vi "Efficiency and Load regulation UI.vi"() -> ()   [LabVIEW 2021]
panel:
  in  "MeasGraphs":T1(tab)
  out "EfficiencyGraph":T2(graph)
  out "LoadRegulationGraph(V/A)":T3(graph)
  out "LoadRegulationGraph(%)":T4(graph)
  out "Load voltage deviation":dbl[](array[numeric])
  out "Load voltages":dbl[](array[numeric])
  out "Efficiency":dbl[](array[numeric])
  out "Load currents":dbl[](array[numeric])
  in  "Source resource name":string caption="RESOURCE NAME"
  in  "Load resource name":string caption="RESOURCE NAME"
  in  "Load Current":dbl
  in  "Source Voltage":dbl
  in  "Load sense":i32(ring)=1009 caption="SENSE" items=["Local"=1008, "Remote"=1009]
  in  "Source sense":i32(ring)=1009 caption="SENSE" items=["Local"=1008, "Remote"=1009]
  out "Status":string
  in  "ELOADResourceName":refnum<k15> caption="RESOURCE NAME"
  in  "PPSResourceName":refnum<k15> caption="RESOURCE NAME"
  in  "DUT setup time":dbl=1.0 caption="DUT SETUP TIME" format="%#_6ps"
  in  "Aperture time":dbl=0.005 caption="APERTURE TIME" format="%#_6ps"
  in  "Source delay":dbl=0.005 caption="SOURCE DELAY" format="%#_6ps"
  in  "Load voltage limit range":dbl=6.0 caption="VOLTAGE LIMIT RANGE" format="%#_6pV"
  in  "Source current limit":dbl=25.0 caption="CURRENT LIMIT" format="%#_6pA"
  in  "Source maximum power":dbl=300.0 caption="MAXIMUM POWER" format="%#_6pW"
  in  "Load configuration":string="Load configuration"
  in  "Source configuration":string="Source configuration"
  in  "Measurement settings":string="Measurement settings"
  in  "Nominal output voltage":dbl=3.3 caption="NOMINAL OUTPUT VOLTAGE" format="%#_6pV"
  in  "Mode of operation":T5(ring)=enum."Perform measurement" caption="MODE OF OPERATION"
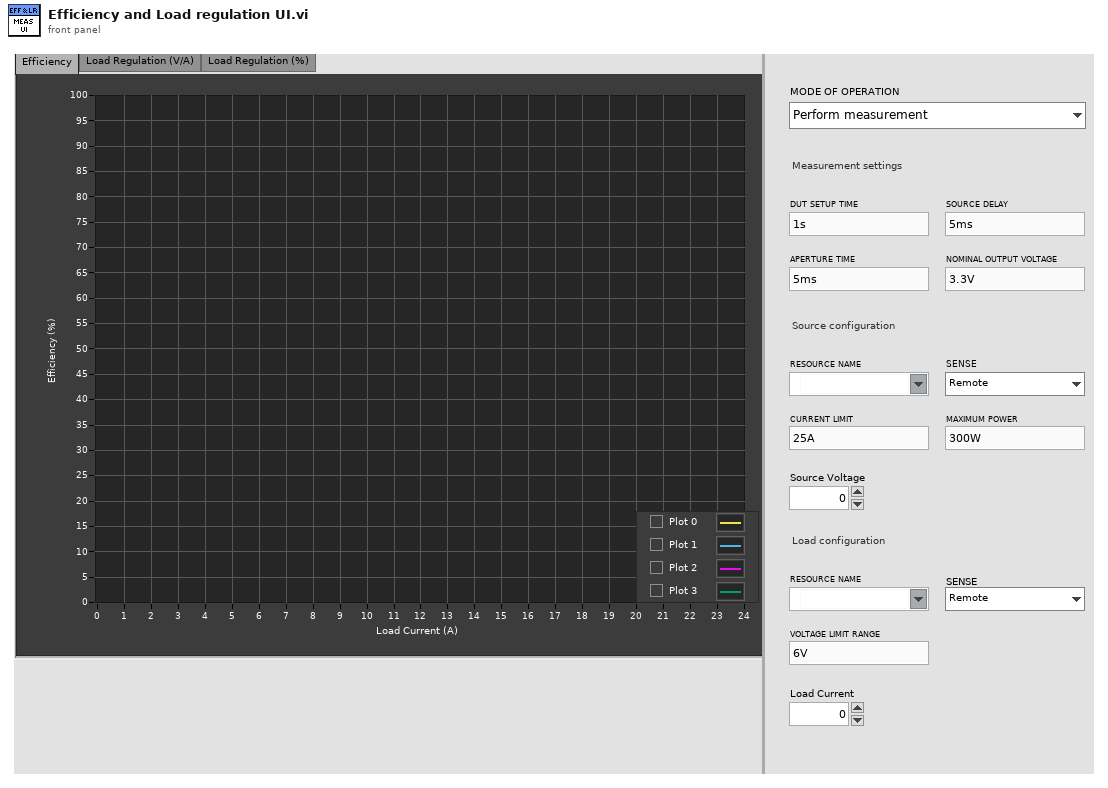
[diagram p1: front panel]
types:
  T1 = enum32{"Efficiency", "Load Regulation (V/A)", "Load Regulation (%)", "Hidden Controls"}
  T2 = cluster{"Load currents":dbl[], "Efficiency":dbl[]}
  T3 = cluster{"Load currents":dbl[], "Load voltages":dbl[]}
  T4 = cluster{"Load currents":dbl[], "Load voltage deviation":dbl[]}
  T5 = enum32{"Power on the DUT", "Perform measurement", "Power off the DUT"}
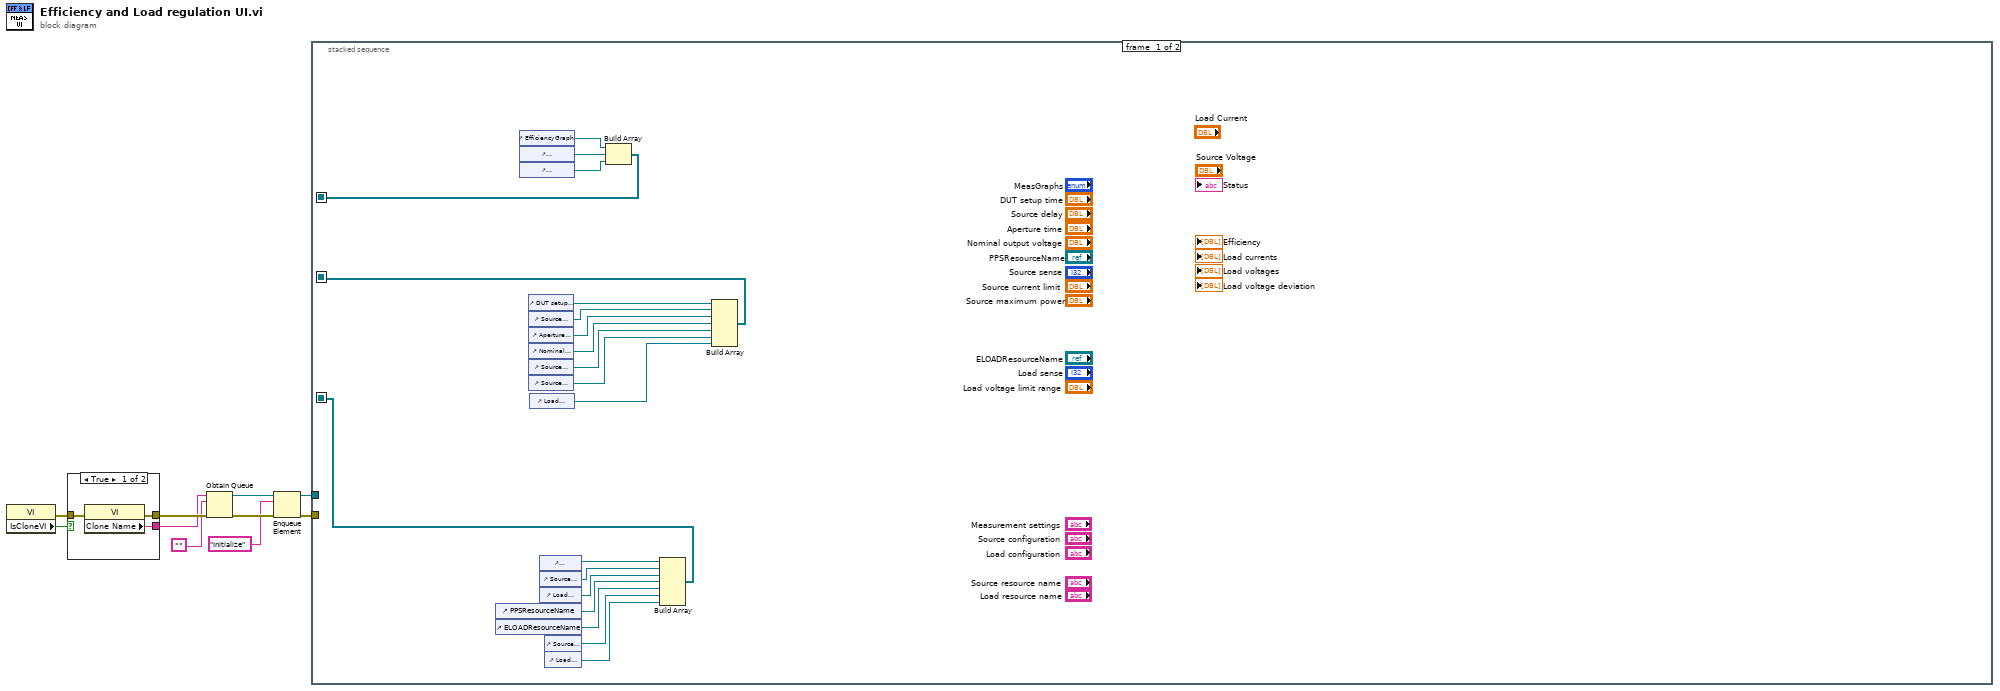
[diagram p0: block diagram]
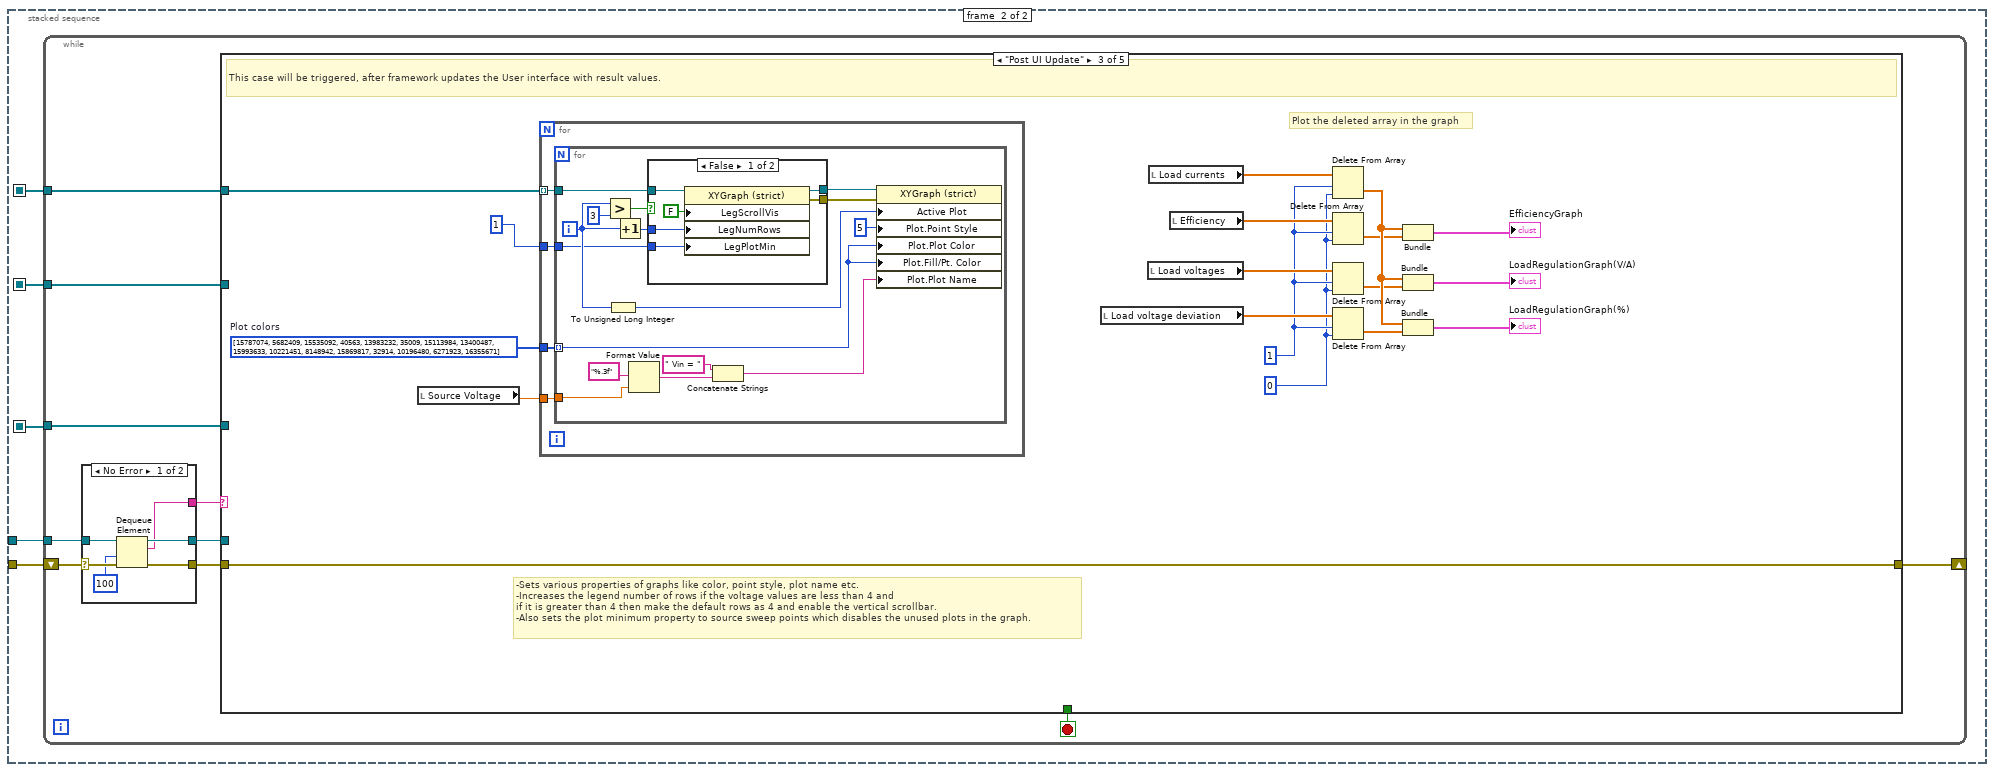
[diagram p2: hidden frame]
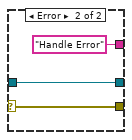
[diagram p3: hidden frame]
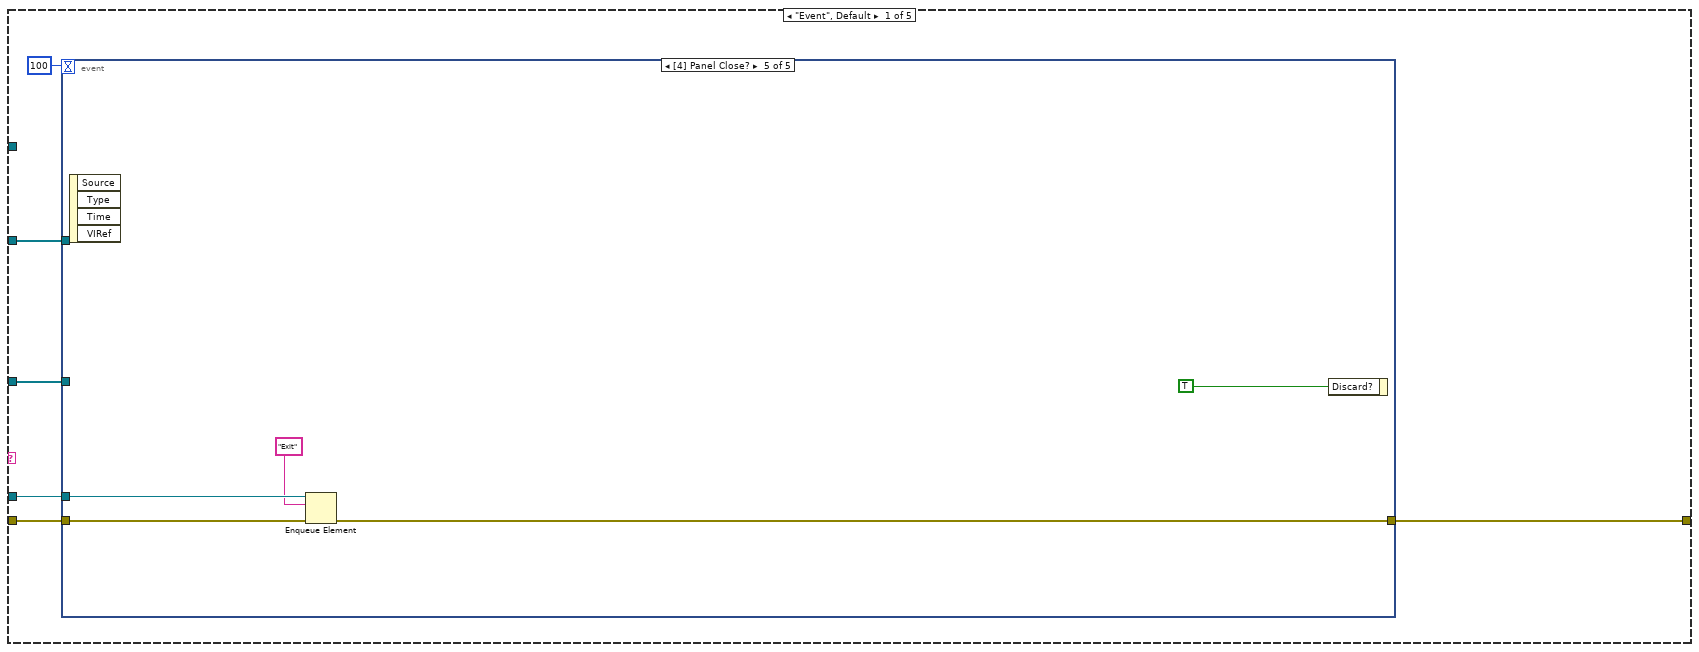
[diagram p4: hidden frame]
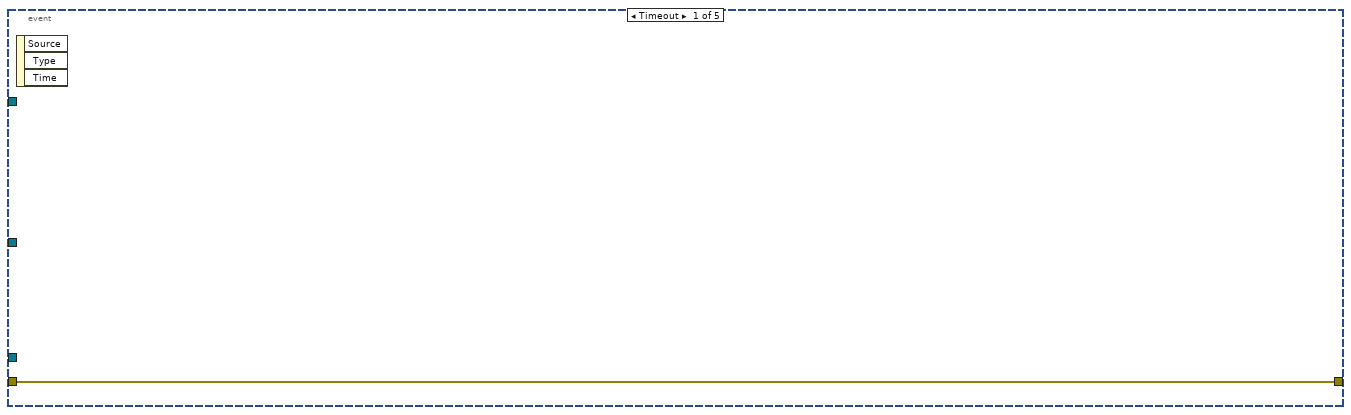
[diagram p5: hidden frame]
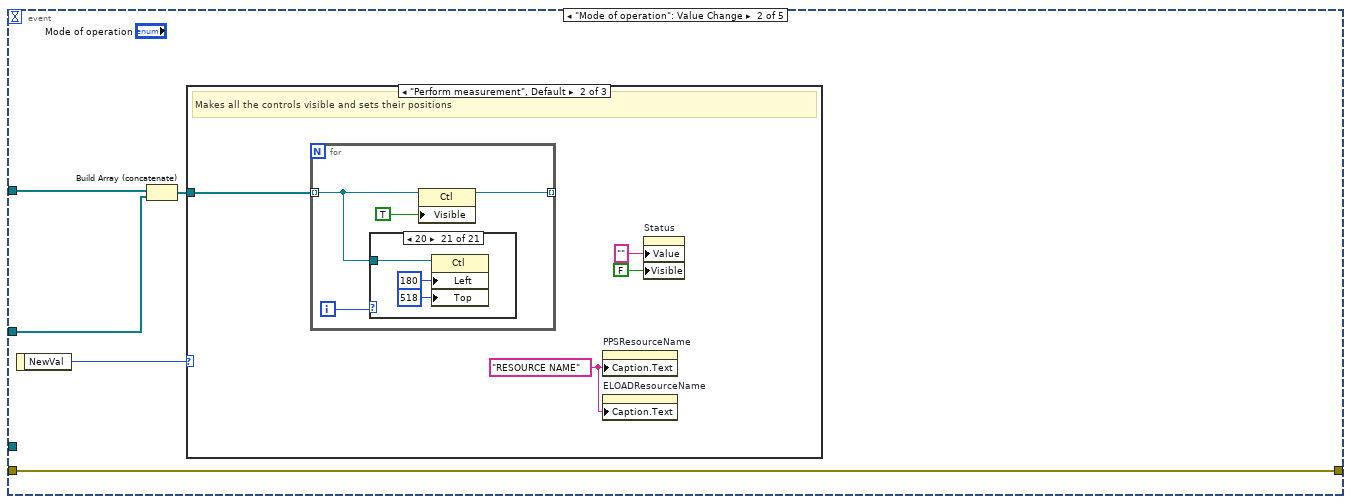
[diagram p6: hidden frame]
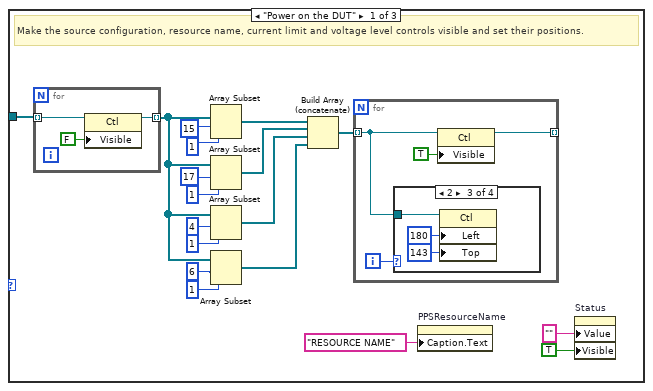
[diagram p7: hidden frame]
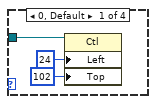
[diagram p8: hidden frame]
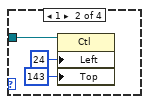
[diagram p9: hidden frame]
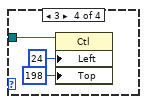
[diagram p10: hidden frame]
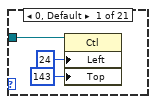
[diagram p11: hidden frame]
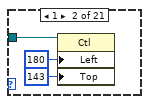
[diagram p12: hidden frame]
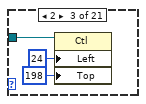
[diagram p13: hidden frame]
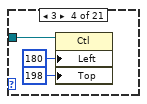
[diagram p14: hidden frame]
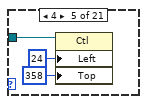
[diagram p15: hidden frame]
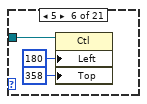
[diagram p16: hidden frame]
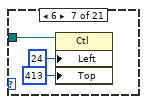
[diagram p17: hidden frame]
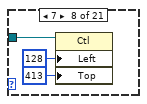
[diagram p18: hidden frame]
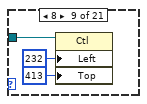
[diagram p19: hidden frame]
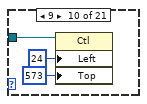
[diagram p20: hidden frame]
diagram:
  n1 = property class="VI"() -> (error out=w1:errorcluster, "IsCloneVI"=w2:bool)  [unwired: 2 in, 1 out]
  n2 = case shown="True" w2 {
    tunnel: [w13 w16] -> w10
    tunnel: [w12 w15] -> w9
    tunnel: w1 -> [w11 w14]
    frame True {
      n3 = property class="VI"(error in=w11) -> (error out=w13:errorcluster, "Clone Name"=w12:string)  [unwired: 1 in, 1 out]
    }
    frame False {
      n4 = property class="VI"(error in=w14) -> (error out=w16:errorcluster, "Name"=w15:string)  [unwired: 1 in, 1 out]
    }
  }
  n5 = Obtain Queue(name (unnamed)=w9, element data type="", error in (no error)=w10) -> (queue out=w6:refnum<queue>, error out=w8:errorcluster)  [unwired: 2 in, 1 out]
  n6 = Enqueue Element(queue=w6, element="Initialize", error in (no error)=w8) -> (queue out=w5:refnum<queue>, error out=w7:errorcluster)  [unwired: 1 in, 1 out]
  n7 = stacked-sequence {
    seq-local: [w19 _] -> [_ w39]
    seq-local: [w20 _] -> [_ w38]
    seq-local: [w21 _] -> [_ w37]
    tunnel: w7 -> [_ w41]
    tunnel: w5 -> [_ w40]
    frame #0 {
      n8 = control-ref of="PPSResourceName"() -> (w26:refnum<vi>)
      n9 = control-ref of="ELOADResourceName"() -> (w25:refnum<vi>)
      n10 = control-ref of="EfficiencyGraph"() -> (w24:refnum<vi>)
      n11 = control-ref of="LoadRegulationGraph(V/A)"() -> (w23:refnum<vi>)
      n12 = control-ref of="LoadRegulationGraph(%)"() -> (w22:refnum<vi>)
      n13 = control-ref of="DUT setup time"() -> (w36:refnum<vi>)
      n14 = control-ref of="Source delay"() -> (w35:refnum<vi>)
      n15 = control-ref of="Aperture time"() -> (w34:refnum<vi>)
      n16 = control-ref of="Nominal output voltage"() -> (w30:refnum<vi>)
      n17 = control-ref of="Source current limit"() -> (w33:refnum<vi>)
      n18 = control-ref of="Source maximum power"() -> (w32:refnum<vi>)
      n19 = control-ref of="Load voltage limit range"() -> (w31:refnum<vi>)
      n20 = control-ref of="Measurement settings"() -> (w29:refnum<vi>)
      n21 = control-ref of="Source configuration"() -> (w27:refnum<vi>)
      n22 = control-ref of="Load configuration"() -> (w28:refnum<vi>)
      n23 = control-ref of="Source sense"() -> (w18:refnum<vi>)
      n24 = control-ref of="Load sense"() -> (w17:refnum<vi>)
      n25 = Build Array(w24, w23, w22) -> (w19:refnum<vi>[])
      n26 = Build Array(w29, w27, w28, w26, w25, w18, w17) -> (w21:refnum<vi>[])
      n27 = Build Array(w36, w35, w34, w30, w33, w32, w31) -> (w20:refnum<vi>[])
    }
    frame #1 {
      n28 = while {
        shift-right: [w46] -> _
        shift-left: w41 -> [w51]
        tunnel: w40 -> [w49]
        tunnel: w38 -> [w44]
        tunnel: w37 -> [w43]
        tunnel: w39 -> [w42]
        stop <- w45 stop-if-true
        n29 = case shown="No Error" w51 {
          selector: w51 -> [w57 w60]
          tunnel: [w56 w60] -> w50
          tunnel: w49 -> [w55 w59]
          tunnel: [w54 w59] -> w48
          tunnel: [w53 "Handle Error"] -> w47
          frame No Error {
            n30 = Dequeue Element(queue=w55, timeout in ms (-1)=100, error in (no error)=w57) -> (queue out=w54:refnum<queue>, element=w53:string, error out=w56:errorcluster)  [unwired: 1 out]
          }
          frame Error {
          }
        }
        n31 = case shown="\"Post UI Update\"" w47 {
          tunnel: w50 -> [w65 w215 w235 w280 w281]
          tunnel: w48 -> [w63 _ _ w278 _]
          tunnel: [w66 w215 w235 w272 w281] -> w46
          tunnel: [_ _ _ TRUE _] -> w45
          tunnel: w44 -> [w62 _ _ w270 _]
          tunnel: w43 -> [w61 _ _ w269 _]
          tunnel: w42 -> [_ w214 w227 w271 _]
          frame "Event", Default {
            n32 = event shown="[4] Panel Close?" {
              selector: _ -> [_ _ _ _ _]
              dyn-events: _ -> [_ _ _ _ _]
              timeout: 100 -> [_ _ _ _ _]
              tunnel: [w67 w68 w203 w205 w209] -> w66
              tunnel: w65 -> [w67 w68 w203 w205 w210]
              tunnel: w63 -> [_ _ _ _ w208]
              tunnel: w62 -> [_ w69 _ _ _]
              tunnel: w61 -> [_ w71 _ _ _]
              event Timeout {
                n33 = event-data() -> ()  [unwired: 1 in, 3 out]
              }
              event "Mode of operation": Value Change {
                n34 = event-data() -> ("NewVal"=w72:T5)  [unwired: 1 in]
                n35 = Build Array (concatenate)(w69, w71) -> (w70:refnum<vi>[])
                n36 = case shown="\"Perform measurement\", Default" w72 {
                  tunnel: w70 -> [w82 w113 w186]
                  frame "Power on the DUT" {
                    # "Make the source configuration, resource name, current limit and voltage level controls visible and set their positions."
                    n37 = for {
                      tunnel: w82 -> [w93] mode=indexing
                      tunnel: [w91] -> w79 mode=indexing
                      n38 = property class="Ctl"(reference=w93, "Visible"=FALSE) -> (reference out=w91:refnum<vi>)  [unwired: 1 in, 1 out]
                    }
                    n39 = Array Subset(array=w79, index=15 ("length"), length=1 ("index")) -> (w81:refnum<vi>[])
                    n40 = Array Subset(array=w79, index=17 ("length"), length=1 ("index")) -> (w80:refnum<vi>[])
                    n41 = Array Subset(array=w79, index=4 ("length"), length=1 ("index")) -> (w78:refnum<vi>[])
                    n42 = Array Subset(array=w79, index=6 ("length"), length=1 ("index")) -> (w76:refnum<vi>[])
                    n43 = Build Array (concatenate)(w81, w80, w78, w76) -> (w77:refnum<vi>[])
                    n44 = for {
                      tunnel: [w96] -> _ mode=indexing
                      tunnel: w77 -> [w94] mode=indexing
                      i -> [w95]
                      n45 = case shown="2" w95 {
                        tunnel: w94 -> [w100 w103 w106 w109]
                        frame 0, Default {
                          n46 = property class="Ctl"(reference=w100, "Left"=24 ("Position:Left"), "Top"=102 ("Position:Top")) -> ()  [unwired: 1 in, 2 out]
                        }
                        frame 1 {
                          n47 = property class="Ctl"(reference=w103, "Left"=24 ("Position:Left"), "Top"=143 ("Position:Top")) -> ()  [unwired: 1 in, 2 out]
                        }
                        frame 2 {
                          n48 = property class="Ctl"(reference=w106, "Left"=180 ("Position:Left"), "Top"=143 ("Position:Top")) -> ()  [unwired: 1 in, 2 out]
                        }
                        frame 3 {
                          n49 = property class="Ctl"(reference=w109, "Left"=24 ("Position:Left"), "Top"=198 ("Position:Top")) -> ()  [unwired: 1 in, 2 out]
                        }
                      }
                      n50 = property class="Ctl"(reference=w94, "Visible"=TRUE) -> (reference out=w96:refnum<vi>)  [unwired: 1 in, 1 out]
                    }
                    n51 = property on="PPSResourceName" class="IVIName"("Caption.Text"="RESOURCE NAME") -> ()  [unwired: 2 in, 2 out]
                    n52 = property on="Status" class="Str"("Value"="" ("Status"), "Visible"=TRUE) -> ()  [unwired: 2 in, 2 out]
                  }
                  frame "Perform measurement", Default {
                    w112 = "RESOURCE NAME" ("Caption.Text")
                    # "Makes all the controls visible and sets their positions"
                    n53 = for {
                      tunnel: w113 -> [w114] mode=indexing
                      tunnel: [w116] -> _ mode=indexing
                      i -> [w115]
                      n54 = case shown="20" w115 {
                        tunnel: w114 -> [w120 w123 w126 w129 w132 w135 w138 w141 w144 w147 w150 w153 w156 w159 w162 w165 w168 w171 w174 w175 w178]
                        frame 0, Default {
                          n55 = property class="Ctl"(reference=w120, "Left"=24 ("Position:Left"), "Top"=143 ("Position:Top")) -> ()  [unwired: 1 in, 2 out]
                        }
                        frame 1 {
                          n56 = property class="Ctl"(reference=w123, "Left"=180 ("Position:Left"), "Top"=143 ("Position:Top")) -> ()  [unwired: 1 in, 2 out]
                        }
                        frame 2 {
                          n57 = property class="Ctl"(reference=w126, "Left"=24 ("Position:Left"), "Top"=198 ("Position:Top")) -> ()  [unwired: 1 in, 2 out]
                        }
                        frame 3 {
                          n58 = property class="Ctl"(reference=w129, "Left"=180 ("Position:Left"), "Top"=198 ("Position:Top")) -> ()  [unwired: 1 in, 2 out]
                        }
                        frame 4 {
                          n59 = property class="Ctl"(reference=w132, "Left"=24 ("Position:Left"), "Top"=358 ("Position:Top")) -> ()  [unwired: 1 in, 2 out]
                        }
                        frame 5 {
                          n60 = property class="Ctl"(reference=w135, "Left"=180 ("Position:Left"), "Top"=358 ("Position:Top")) -> ()  [unwired: 1 in, 2 out]
                        }
                        frame 6 {
                          n61 = property class="Ctl"(reference=w138, "Left"=24 ("Position:Left"), "Top"=413 ("Position:Top")) -> ()  [unwired: 1 in, 2 out]
                        }
                        frame 7 {
                          n62 = property class="Ctl"(reference=w141, "Left"=128 ("Position:Left"), "Top"=413 ("Position:Top")) -> ()  [unwired: 1 in, 2 out]
                        }
                        frame 8 {
                          n63 = property class="Ctl"(reference=w144, "Left"=232 ("Position:Left"), "Top"=413 ("Position:Top")) -> ()  [unwired: 1 in, 2 out]
                        }
                        frame 9 {
                          n64 = property class="Ctl"(reference=w147, "Left"=24 ("Position:Left"), "Top"=573 ("Position:Top")) -> ()  [unwired: 1 in, 2 out]
                        }
                        frame 10 {
                          n65 = property class="Ctl"(reference=w150, "Left"=180 ("Position:Left"), "Top"=573 ("Position:Top")) -> ()  [unwired: 1 in, 2 out]
                        }
                        frame 11 {
                          n66 = property class="Ctl"(reference=w153, "Left"=24 ("Position:Left"), "Top"=628 ("Position:Top")) -> ()  [unwired: 1 in, 2 out]
                        }
                        frame 12 {
                          n67 = property class="Ctl"(reference=w156, "Left"=128 ("Position:Left"), "Top"=628 ("Position:Top")) -> ()  [unwired: 1 in, 2 out]
                        }
                        frame 13 {
                          n68 = property class="Ctl"(reference=w159, "Left"=232 ("Position:Left"), "Top"=628 ("Position:Top")) -> ()  [unwired: 1 in, 2 out]
                        }
                        frame 14 {
                          n69 = property class="Ctl"(reference=w162, "Left"=24 ("Position:Left"), "Top"=102 ("Position:Top")) -> ()  [unwired: 1 in, 2 out]
                        }
                        frame 15 {
                          n70 = property class="Ctl"(reference=w165, "Left"=24 ("Position:Left"), "Top"=262 ("Position:Top")) -> ()  [unwired: 1 in, 2 out]
                        }
                        frame 16 {
                          n71 = property class="Ctl"(reference=w168, "Left"=24 ("Position:Left"), "Top"=477 ("Position:Top")) -> ()  [unwired: 1 in, 2 out]
                        }
                        frame 17 {
                          n72 = property class="Ctl"(reference=w171, "Left"=24 ("Position:Left"), "Top"=303 ("Position:Top")) -> ()  [unwired: 1 in, 2 out]
                        }
                        frame 18 {
                          n73 = property class="Ctl"(reference=w174, "Left"=24 ("Position:Left"), "Top"=518 ("Position:Top")) -> ()  [unwired: 1 in, 2 out]
                        }
                        frame 19 {
                          n74 = property class="Ctl"(reference=w175, "Left"=180 ("Position:Left"), "Top"=303 ("Position:Top")) -> ()  [unwired: 1 in, 2 out]
                        }
                        frame 20 {
                          n75 = property class="Ctl"(reference=w178, "Left"=180 ("Position:Left"), "Top"=518 ("Position:Top")) -> ()  [unwired: 1 in, 2 out]
                        }
                      }
                      n76 = property class="Ctl"(reference=w114, "Visible"=TRUE) -> (reference out=w116:refnum<vi>)  [unwired: 1 in, 1 out]
                    }
                    n77 = property on="PPSResourceName" class="IVIName"("Caption.Text"=w112) -> ()  [unwired: 2 in, 2 out]
                    n78 = property on="ELOADResourceName" class="IVIName"("Caption.Text"=w112) -> ()  [unwired: 2 in, 2 out]
                    n79 = property on="Status" class="Str"("Value"="" ("Status"), "Visible"=FALSE) -> ()  [unwired: 2 in, 2 out]
                  }
                  frame "Power off the DUT" {
                    # "Makes only the Source and Load Resource Name controls visible and sets their positions"
                    n80 = for {
                      tunnel: w186 -> [w191] mode=indexing
                      tunnel: [w190] -> w185 mode=indexing
                      n81 = property class="Ctl"(reference=w191, "Visible"=FALSE) -> (reference out=w190:refnum<vi>)  [unwired: 1 in, 1 out]
                    }
                    n82 = Array Subset(array=w185, index=17 ("length"), length=2 ("index")) -> (w187:refnum<vi>[])
                    n83 = property on="PPSResourceName" class="IVIName"("Caption.Text"="SOURCE RESOURCE NAME") -> ()  [unwired: 2 in, 2 out]
                    n84 = property on="ELOADResourceName" class="IVIName"("Caption.Text"="LOAD RESOURCE NAME") -> ()  [unwired: 2 in, 2 out]
                    n85 = for {
                      tunnel: w187 -> [w193] mode=indexing
                      tunnel: [w195] -> _ mode=indexing
                      i -> [w194]
                      n86 = case shown="0, Default" w194 {
                        tunnel: w193 -> [w199 w202]
                        frame 0, Default {
                          n87 = property class="Ctl"(reference=w199, "Left"=24 ("Position:Left"), "Top"=102 ("Position:Top")) -> ()  [unwired: 1 in, 2 out]
                        }
                        frame 1 {
                          n88 = property class="Ctl"(reference=w202, "Left"=24 ("Position:Left"), "Top"=157 ("Position:Top")) -> ()  [unwired: 1 in, 2 out]
                        }
                      }
                      n89 = property class="Ctl"(reference=w193, "Visible"=TRUE) -> (reference out=w195:refnum<vi>)  [unwired: 1 in, 1 out]
                    }
                    n90 = property on="Status" class="Str"("Value"="" ("Status"), "Visible"=TRUE) -> ()  [unwired: 2 in, 2 out]
                  }
                }
              }
              event "PPSResourceName": Value Change {
                n91 = event-data() -> ()  [unwired: 1 in, 1 out]
                n92 = property on="PPSResourceName" class="IVIName"() -> ("Value"=w204:refnum<k15>)  [unwired: 2 in, 2 out]
                n93 = property on="Source resource name" class="Str"("Value"=w204) -> ()  [unwired: 2 in, 2 out]
              }
              event "ELOADResourceName": Value Change {
                n94 = event-data() -> ()  [unwired: 1 in, 1 out]
                n95 = property on="ELOADResourceName" class="IVIName"() -> ("Value"=w206:refnum<k15>)  [unwired: 2 in, 2 out]
                n96 = property on="Load resource name" class="Str"("Value"=w206) -> ()  [unwired: 2 in, 2 out]
              }
              event Panel Close? {
                n97 = event-data() -> ()  [unwired: 1 in, 4 out]
                n98 = Enqueue Element(queue=w208, element="Exit", error in (no error)=w210) -> (error out=w209:errorcluster)  [unwired: 1 in, 2 out]
                n99 = event-data("Discard?"=TRUE) -> ()  [unwired: 1 in, 1 out]
              }
            }
          }
          frame "Initialize" {
            w213 = "<Select Device>"
            n100 = for {
              tunnel: w214 -> [w216] mode=indexing
              n101 = property class="XYGraph (strict)"(reference=w216, "ActPaletteTool"=2 ("Palette:Active Tool")) -> ()  [unwired: 1 in, 2 out]
            }
            n102 = property on="PPSResourceName" class="IVIName"("Value"=w213) -> ()  [unwired: 2 in, 2 out]
            n103 = property on="ELOADResourceName" class="IVIName"("Value"=w213) -> ()  [unwired: 2 in, 2 out]
            n104 = property on="Status" class="Str"("Visible"=FALSE) -> ()  [unwired: 2 in, 2 out]
          }
          frame "Post UI Update" {
            w219 = 0 ("index")
            w224 = 1 ("Load sweep points")
            w226 = u32[] [15787074, 5682409, 15535092, 40563, 13983232, 35009, 15113984, 13400487, 15993633, 10221451, 8148942, 15869817, 32914, 10196480, 6271923, 16355671]  # Plot colors
            # "-Sets various properties of graphs like color, point style, plot name etc.\n-Increases the legend number of rows if the voltage values are less than 4 and \nif it is greater than 4 then make the default rows as 4 and enable the vertical scrollbar.\n-Also sets the plot minimum property to source sweep points which disables the unused plots in the graph."
            # "Plot the deleted array in the graph"
            # "This case will be triggered, after framework updates the User interface with result values."
            n105 = local read "Source Voltage"() -> (w225:dbl)
            n106 = for {
              tunnel: w225 -> [w239]
              tunnel: w227 -> [w238] mode=indexing
              tunnel: 1 ("y") -> [w237]
              tunnel: w226 -> [w236]
              n107 = for {
                tunnel: w239 -> [w252]
                tunnel: w238 -> [w245]
                tunnel: w237 -> [w242]
                tunnel: w236 -> [w248] mode=indexing
                i -> [w246]
                n108 = Greater?(x=w246, y=3) -> (0:w250:bool)
                n109 = To Unsigned Long Integer(number=w246) -> (unsigned 32bit integer=w249:u32)
                n110 = Increment(x=w246) -> (x+1=w244:i32)
                n111 = Format Value(format string="%.3f", value (0)=w252) -> (output string=w255:string)  [unwired: 1 out]
                n112 = case shown="False" w250 {
                  tunnel: w245 -> [w261 w267]
                  tunnel: w244 -> [w260 _]
                  tunnel: [w259 w266] -> w243
                  tunnel: w242 -> [w257 w262]
                  tunnel: [w258 w265] -> w241
                  frame False {
                    n113 = property on="Property Node" class="XYGraph (strict)"(reference=w261, "LegScrollVis"=FALSE ("Legend:Scrollbar Visible"), "LegNumRows"=w260, "LegPlotMin"=w257) -> (reference out=w259:refnum<vi>, error out=w258:errorcluster)  [unwired: 1 in]
                  }
                  frame True {
                    n114 = property on="Property Node" class="XYGraph (strict)"(reference=w267, "LegScrollVis"=TRUE ("Legend:Scrollbar Visible"), "LegNumRows"=u32 4 ("Legend:Number of Rows"), "LegPlotMin"=w262) -> (reference out=w266:refnum<vi>, error out=w265:errorcluster)  [unwired: 1 in]
                  }
                }
                n115 = Concatenate Strings(" Vin = " ("string"), w255) -> (w240:string)
                n116 = property on="Property Node" class="XYGraph (strict)"(reference=w243, error in=w241, "Active Plot"=w249, "Plot.Point Style"=u8 5, "Plot.Plot Color"=w248, "Plot.Fill/Pt. Color"=w248, "Plot.Plot Name"=w240) -> ()  [unwired: 2 out]
              }
            }
            n117 = local read "Load voltage deviation"() -> (w234:dbl[])
            n118 = local read "Load voltages"() -> (w233:dbl[])
            n119 = local read "Load currents"() -> (w232:dbl[])
            n120 = local read "Efficiency"() -> (w231:dbl[])
            n121 = Delete From Array(array=w232, length=w224, index=w219) -> (deleted portion=w223:dbl[])  [unwired: 1 out]
            n122 = Delete From Array(array=w231, length=w224, index=w219) -> (deleted portion=w220:dbl[])  [unwired: 1 out]
            n123 = Delete From Array(array=w233, length=w224, index=w219) -> (deleted portion=w221:dbl[])  [unwired: 1 out]
            n124 = Delete From Array(array=w234, length=w224, index=w219) -> (deleted portion=w222:dbl[])  [unwired: 1 out]
            n125 = Bundle("Load currents"=w223, "Efficiency"=w220) -> (→"EfficiencyGraph":T2)  [unwired: 1 in]
            n126 = Bundle("Load currents"=w223, "Load voltages"=w221) -> (→"LoadRegulationGraph(V/A)":T3)  [unwired: 1 in]
            n127 = Bundle("Load currents"=w223, "Load voltage deviation"=w222) -> (→"LoadRegulationGraph(%)":T4)  [unwired: 1 in]
          }
          frame "Exit" {
            # "This case is triggered to close the User Interface from framework"
            n128 = Build Array (concatenate)(w271, w270, w269) -> (w268:refnum<vi>[])
            n129 = Close Reference(reference=w268) -> (error out=w274:errorcluster)  [unwired: 1 in]
            n130 = Flush Queue(queue=w278, error in (no error)=w280) -> (queue out=w277:refnum<queue>, error out=w276:errorcluster)  [unwired: 1 out]
            n131 = Release Queue(queue=w277, force destroy? (F)=TRUE, error in (no error)=w276) -> (error out=w273:errorcluster)  [unwired: 2 out]
            n132 = Merge Errors(w274, w273) -> (w272:errorcluster)
          }
          frame "Handle Error" {
          }
        }
      }
    }
  }
